vi "rs3 set advanced mode.vi"(8 "error in (no error)":errorcluster, 10 "enable":i32, 11 "device in":u64) -> (0 "error out":errorcluster, 1 "error":u64, 3 "device out":u64)   [LabVIEW 2018, in "libRealSense3.lvlib"]
doc: "Enables or disables the Advanced Mode. If the device is NOT in Advanced mode then the advanced depth and color commands will not work. HOWEVER, setting Advanced mode may restart the device. \nThis mode persists, even after unplugging the device. \n\nINPUT:\nDev in Input device\nEnable Enable=1 is on. \n\nOUTPUT:\nerror error=0 is no error"
uses:
  libRealSense3.lvlib
  realsense2.dll
panel:
  # "RS3 Set Advanced Mode"
  # "(C) 2017 Intel Corp.,  AGJ"
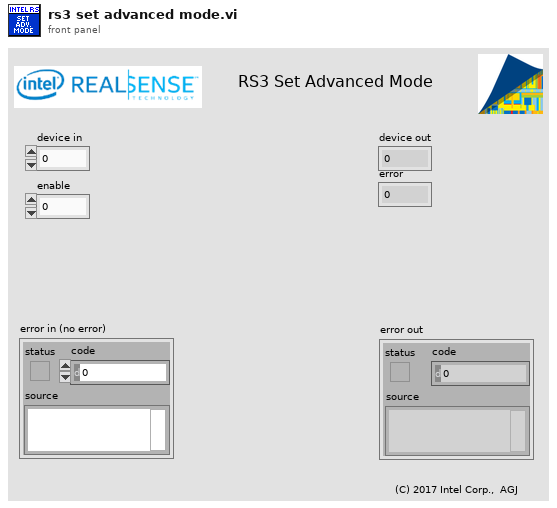
[diagram p1: front panel]
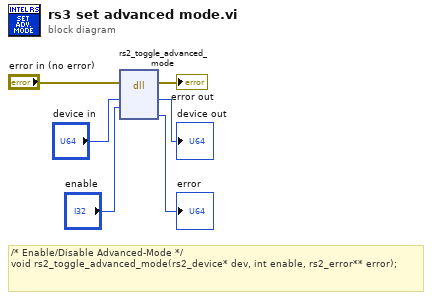
[diagram p0: block diagram]
diagram:
  # "/* Enable/Disable Advanced-Mode */\nvoid rs2_toggle_advanced_mode(rs2_device* dev, int enable, rs2_error** error);"
  n1 = dll-call lib="C:/Users/aaron.jencks/Documents/Temp/realsense_labview_sdk/RealSense SDK2.11.0 for LabVIEW/realsense2.dll" fn="rs2_toggle_advanced_mode"(error in="error in (no error)", "device in"="device in", "enable"="enable") -> (error out=→"error out":errorcluster, "device in"=→"device out":u64, "error"=→"error":u64)  [unwired: 5 in, 1 out]
